vi "[X] ~ 0 [DBL].vi"(1 "Tolerance (1E-6)":dbl=1e-06, 7 "X":dbl[](array[numeric]) format="%#_9g") -> (8 "~ 0 ?":bool[](array[boolean]))   [LabVIEW 2021, in "Comparison.lvlib"]
uses:
  Comparison.lvlib
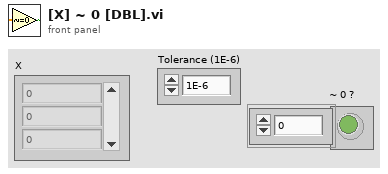
[diagram p1: front panel]
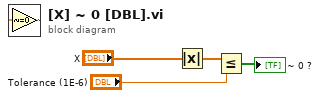
[diagram p0: block diagram]
diagram:
  n1 = Absolute Value(x="X") -> (abs(x)=w1:dbl[])
  n2 = Less Or Equal?(x=w1, y="Tolerance (1E-6)") -> (x <= y?=→"~ 0 ?":bool[])
